vi "prepAO_sealtest.vi"(1 "Vhold":dbl, 2 "samples per channel":i32=1000) -> ()   [LabVIEW 2015]
uses:
  <vilib>/DAQmx/write.llb/DAQmx Write (Analog 1D Wfm NChan NSamp).vi
  <vilib>/DAQmx/create/channels.llb/DAQmx Create Channel (AO-Voltage-Basic).vi
  <vilib>/DAQmx/configure/timing.llb/DAQmx Timing (Sample Clock).vi
  <vilib>/DAQmx/miscellaneous.llb/DAQmx Fill In Error Info.vi
  <vilib>/DAQmx/configure/trigger.llb/DAQmx Start Trigger (Digital Edge).vi
panel:
  out "number of samples written per channel":u32
  in  "error in 2":errorcluster caption="error in"
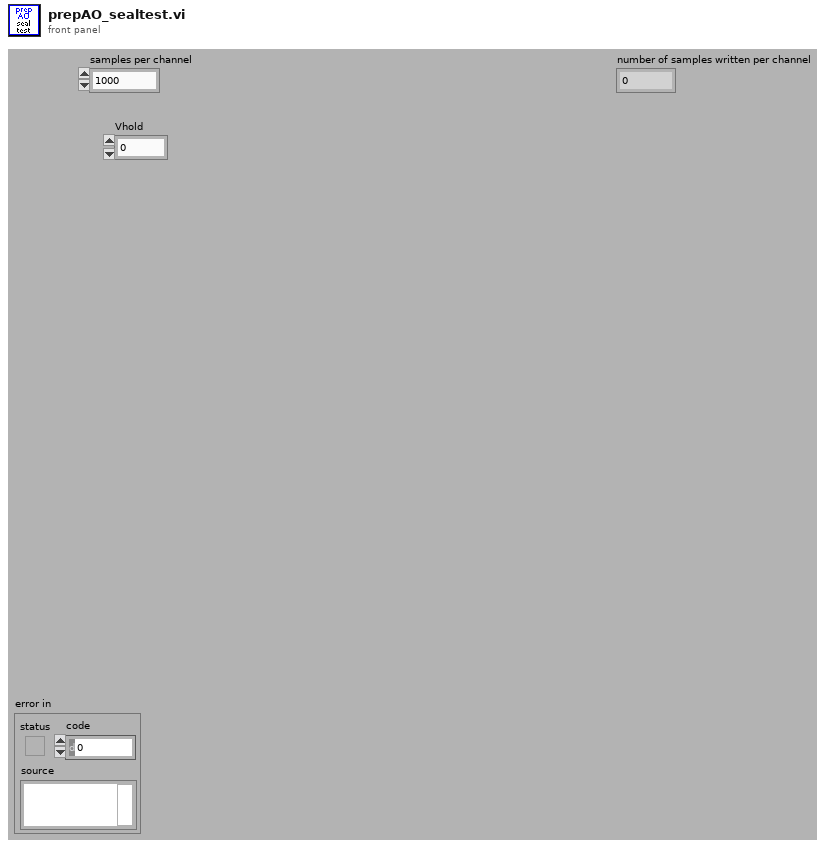
[diagram p1: front panel]
types:
  T1 = cluster{"StageS":i32, "StageL":i32, "currmeas data dir":path, "image OD":u16, "contour OD":u16, "point OD":u16, "AOlines":tag[], "AIlines":tag[], "CI lines":tag[], "DO lines":tag[], "AO names":string[], "CI names":string[], "AI names":string[], "DO names":string[], "CIextensions":string[], "AIextensions":string[], "Voltage to Ygalvo":i32, "Voltage to Xgalvo":i32, "Voltage to patch":i32, "640 shutter":i32, "2P shutter":i32, "LT timestamp":u32, "Vp":i32, "Ip":i32, "camera trigger":i32, "master data dir":path, "voltage to Zpos":i32, "Vto2P":i32, "640 AO":i32, "488 AO":i32, "532 AO":i32, "640TTL":u32, "488TTL":u32, "532TTL":u32, "Device 1 sampleclock out":tag, "Device 1 Starttrigger out":tag, "Device 2 sampleclock in":tag, "Device 2 StartTrigger in ":tag, "2PODTTL":u32, "488 shutter":u32, "LCVR red":u32, "LCVR blue":u32}
  T2 = cluster{"AO parameters":cluster{"AOtab":dbl, "Repeats":dbl, "Cycles":dbl, "Start amplitude (V)":dbl, "Baseline (V)":dbl, "Step size (V)":dbl, "DC (%)":dbl, "Sampling frequency (Hz)":dbl, "Period (ms)":dbl, "Offset (V)":dbl, "Amplitude (V)":dbl, "Frequency":dbl, "Tri Repeats":dbl, "Cycle length (s)":dbl, "Pulses":dbl, "Matlab wave file":path, "Tri phase":dbl, "padding value":dbl}[]}
  T3 = cluster{"AOtab":dbl, "Repeats":dbl, "Cycles":dbl, "Start amplitude (V)":dbl, "Baseline (V)":dbl, "Step size (V)":dbl, "DC (%)":dbl, "Sampling frequency (Hz)":dbl, "Period (ms)":dbl, "Offset (V)":dbl, "Amplitude (V)":dbl, "Frequency":dbl, "Tri Repeats":dbl, "Cycle length (s)":dbl, "Pulses":dbl, "Matlab wave file":path, "Tri phase":dbl, "padding value":dbl}[]
  T4 = cluster{"AOtab":dbl, "Repeats":dbl, "Cycles":dbl, "Start amplitude (V)":dbl, "Baseline (V)":dbl, "Step size (V)":dbl, "DC (%)":dbl, "Sampling frequency (Hz)":dbl, "Period (ms)":dbl, "Offset (V)":dbl, "Amplitude (V)":dbl, "Frequency":dbl, "Tri Repeats":dbl, "Cycle length (s)":dbl, "Pulses":dbl, "Matlab wave file":path, "Tri phase":dbl, "padding value":dbl}
  T5 = cluster{"AO":refnum<k21>[], "E_AO":errorcluster[]}
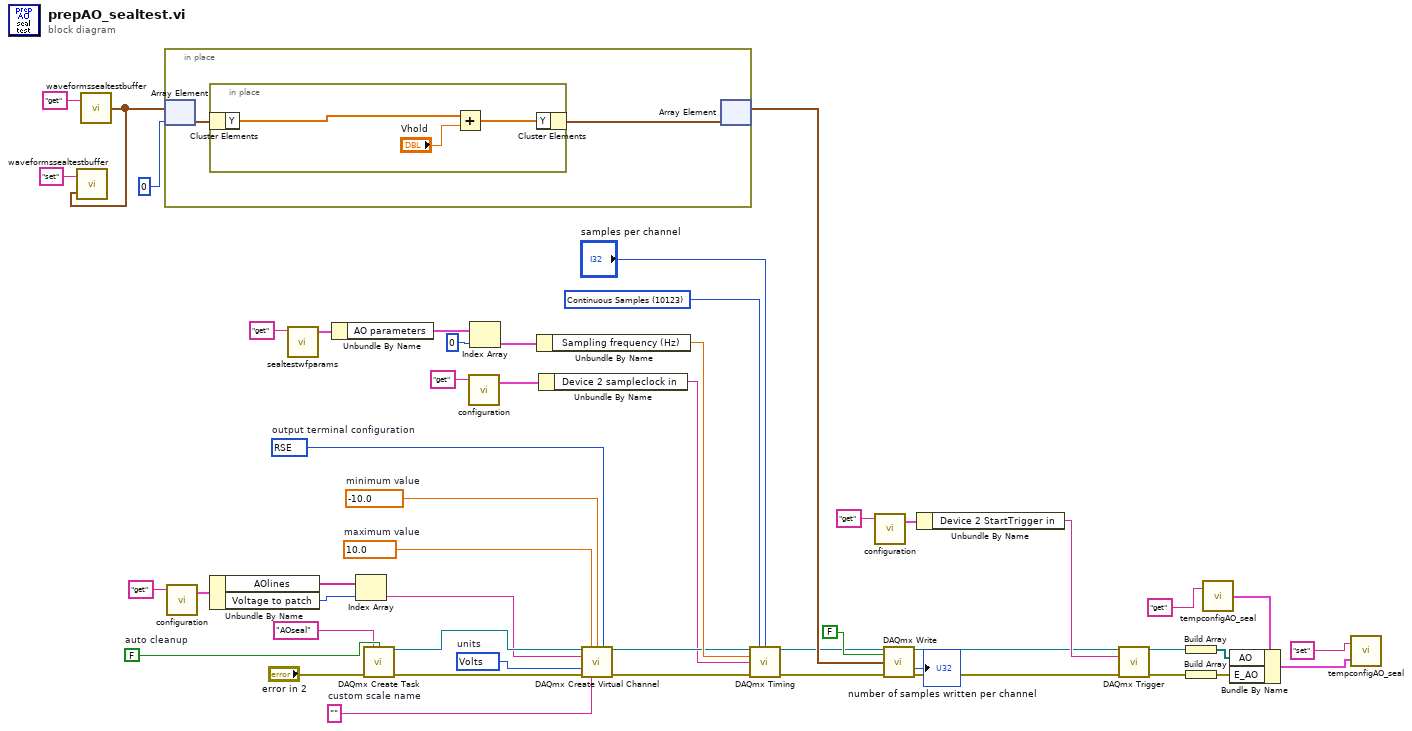
[diagram p0: block diagram]
diagram:
  w27 = 10123 items=["Finite Samples"=10178, "Continuous Samples"=10123, "Hardware Timed Single Point"=12522] ("sample mode")
  w43 = 10083 items=["Default"=-1, "RSE"=10083, "Differential"=10106, "Pseudodifferential"=12529]  # output terminal configuration
  w42 = 10348 items=["Volts"=10348, "From Custom Scale"=10065]  # units
  w35 = ""  # custom scale name
  w41 = -10.0  # minimum value
  w40 = 10.0  # maximum value
  w48 = FALSE  # auto cleanup
  n1 = call "waveformssealtestbuffer.vi"("command"="get") -> ("AO wf out"=w5:waveform(dbl)[])  [unwired: 1 in]
  n2 = call "waveformssealtestbuffer.vi"("AO wf in"=w5, "command"="set") -> ()  [unwired: 1 out]
  n3 = in-place {
    n4 = in-place-array #1(w5, 0) -> (w52:waveform(dbl))
    n5 = in-place {
      n6 = in-place-cluster #2(w52) -> ("Y"=w55:dbl[])
      n7 = Add(x=w55, y="Vhold") -> (x+y=w54:dbl[])
      n8 = in-place-cluster #2("Y"=w54) -> (w51:waveform(dbl))
    }
    n9 = in-place-array #1(w51) -> (w24:waveform(dbl)[])  [unwired: 1 out]
  }
  n10 = call "configuration.vi"("command"="get") -> ("config out"=w37:T1)  [unwired: 2 in, 1 out]
  n11 = Unbundle By Name(w37) -> ("AOlines"=w39:tag[], "Voltage to patch"=w34:i32)
  n12 = call "sealtestwfparams.vi"("command"="get") -> ("Params out"=w32:T2)  [unwired: 6 in]
  n13 = Unbundle By Name(w32) -> ("AO parameters"=w30:T3)
  n14 = Index Array(array=w39, index=w34) -> (element=w36:tag)
  n15 = call <vilib>:"DAQmx Create Task.vi"("new task name"="AOseal", "auto cleanup"=w48, "error in"="error in 2") -> ("task out"=w49:refnum<k21>, "error out"=w50:errorcluster)  [unwired: 11 in]
  n16 = call "configuration.vi"("command"="get") -> ("config out"=w18:T1)  [unwired: 2 in, 1 out]
  n17 = Index Array(array=w30, index=0) -> (element=w29:T4)
  n18 = Unbundle By Name(w29) -> ("Sampling frequency (Hz)"=w26:dbl)
  n19 = Unbundle By Name(w18) -> ("Device 2 sampleclock in"=w16:tag)
  n20 = call-poly <vilib>:"DAQmx Create Virtual Channel.vi"("task in"=w49, "maximum value"=w40, "minimum value"=w41, "output terminal configuration"=w43, "physical channels"=w36, "units"=w42, "error in"=w50, "custom scale name"=w35) -> ("task out"=w21:refnum<k21>, "error out"=w20:errorcluster)  [unwired: 6 in]
  n21 = call-poly <vilib>:"DAQmx Timing.vi"("task/channels in"=w21, "sample mode"=w27, "samples per channel"="samples per channel", "rate"=w26, "source"=w16, "error in"=w20) -> ("task out"=w12:refnum<k21>, "error out"=w45:errorcluster)  [unwired: 1 in, 7 out]
  n22 = call "configuration.vi"("command"="get") -> ("config out"=w14:T1)  [unwired: 2 in, 1 out]
  n23 = call-poly <vilib>:"DAQmx Write.vi"("task/channels in"=w12, "auto start"=FALSE, "data"=w24, "error in"=w45) -> ("task out"=w11:refnum<k21>, "number of samples written per channel"=→"number of samples written per channel":u32, "error out"=w9:errorcluster)  [unwired: 9 in]
  n24 = Unbundle By Name(w14) -> ("Device 2 StartTrigger in"=w15:tag)
  n25 = call-poly <vilib>:"DAQmx Trigger.vi"("task/channels in"=w11, "source"=w15, "error in"=w9) -> ("task out"=w10:refnum<k21>, "error out"=w8:errorcluster)  [unwired: 11 in]
  n26 = Build Array(w10) -> (w23:refnum<k21>[])
  n27 = Build Array(w8) -> (w22:errorcluster[])
  n28 = call "tempconfigAO_seal.vi"("command"="get") -> ("Temp Config out"=w3:T5)  [unwired: 1 in]
  n29 = Bundle By Name(cluster=w3, "AO"=w23, "E_AO"=w22) -> (w1:T5)
  n30 = call "tempconfigAO_seal.vi"("Temp Config in"=w1, "command"="set") -> ()  [unwired: 1 out]
